vi "pick_point.vi"(4 "Modelview Matrix":sgl[][](array[numeric]), 6 "Projection Matrix":sgl[][](array[numeric]), 7 "Vertex Array":cluster{"X":sgl, "Y":sgl, "Z":sgl}[](array[cluster]), 8 "Translate By":T2, 9 "Scale By":T2, 10 "Point":cluster{"X":i32, "Y":i32}={"X"=2, "Y"=2}, 11 "ContentBounds":T1) -> (0 "Hit Any Point?":bool, 1 "Actual Ouput Coordinate":T2, 2 "Up Vect":T2, 3 "Forward Vect":T2)   [LabVIEW 2020, in "3DPC_SurfacePlot.xctl"]
uses:
  <vilib>/Native 3D Graph/xcontrol/3DPC_SurfacePlot.xctl
  <vilib>/Native 3D Graph/typedefs/vector.ctl
  <vilib>/Utility/miscctls.llb/LVBoundsTypeDef.ctl
  <vilib>/Analysis/baseanly.llb/A x Vector.vi
  <vilib>/Analysis/baseanly.llb/Real Inverse Matrix.vi
  <vilib>/Analysis/NI_AALBase.lvlib
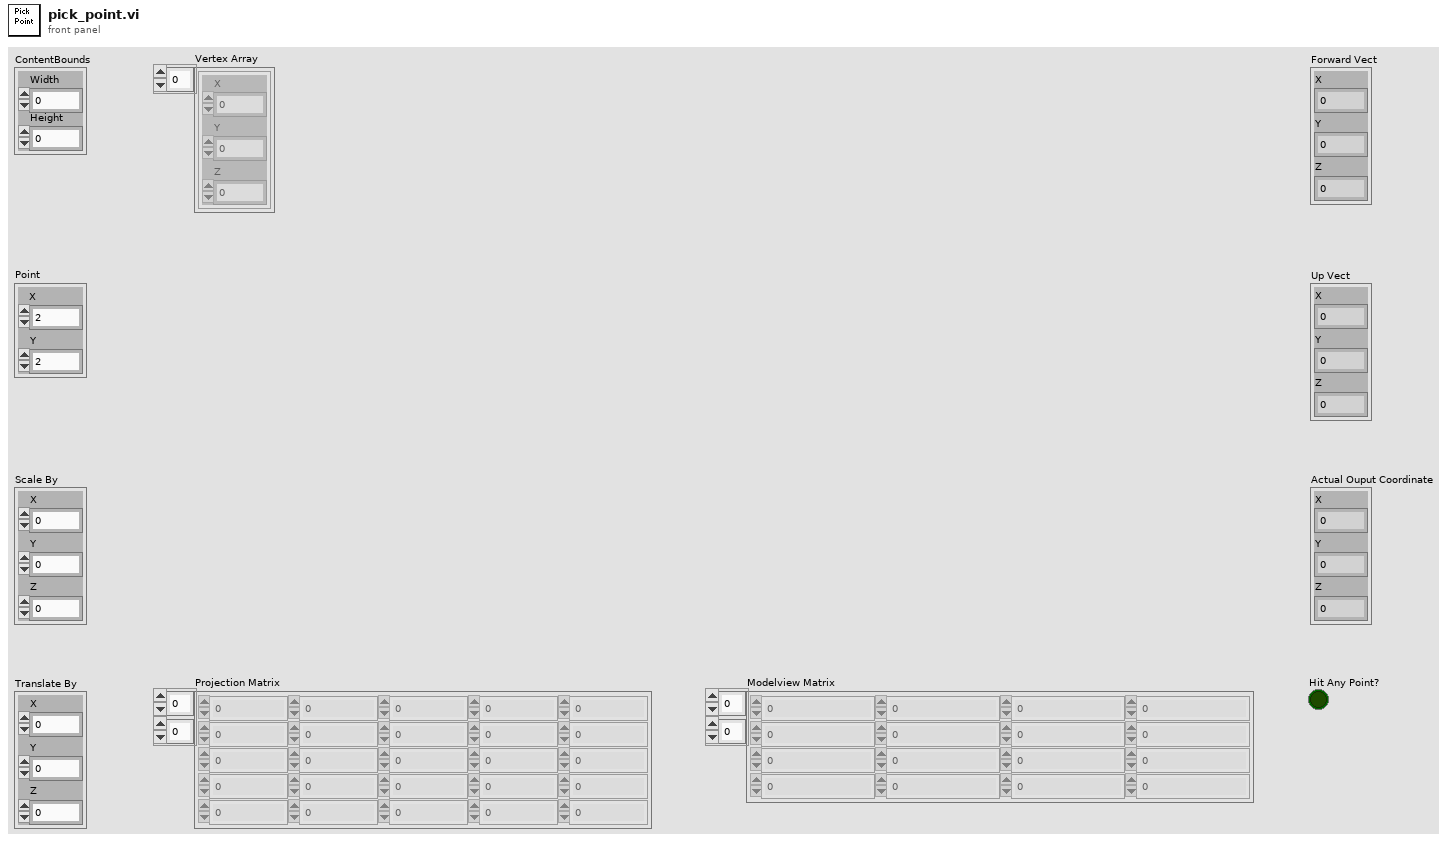
[diagram p1: front panel]
types:
  T1 = typedef "LVBoundsTypeDef.ctl" = cluster{"Width":u32, "Height":u32}
  T2 = typedef "3DPC_SurfacePlot.xctl/vector.ctl" = cluster{"X":sgl, "Y":sgl, "Z":sgl}
  T3 = cluster{"Real Matrix Element":dbl, "Real Matrix Element":dbl, "Real Matrix Element":dbl}[]
  T4 = cluster{"Real Matrix Element":i32, "Real Matrix Element":i32, "Real Matrix Element":i32}
  T5 = typedef "NI_Matrix.lvlib/RealMatrix.ctl" = dbl[][]
  T6 = cluster{"A x Vector[0]":dbl, "A x Vector[1]":dbl, "A x Vector[2]":dbl}
  T7 = cluster{cluster{"A x Vector[0]":dbl, "A x Vector[1]":dbl, "A x Vector[2]":dbl}, cluster{"A x Vector[0]":dbl, "A x Vector[1]":dbl, "A x Vector[2]":dbl}}
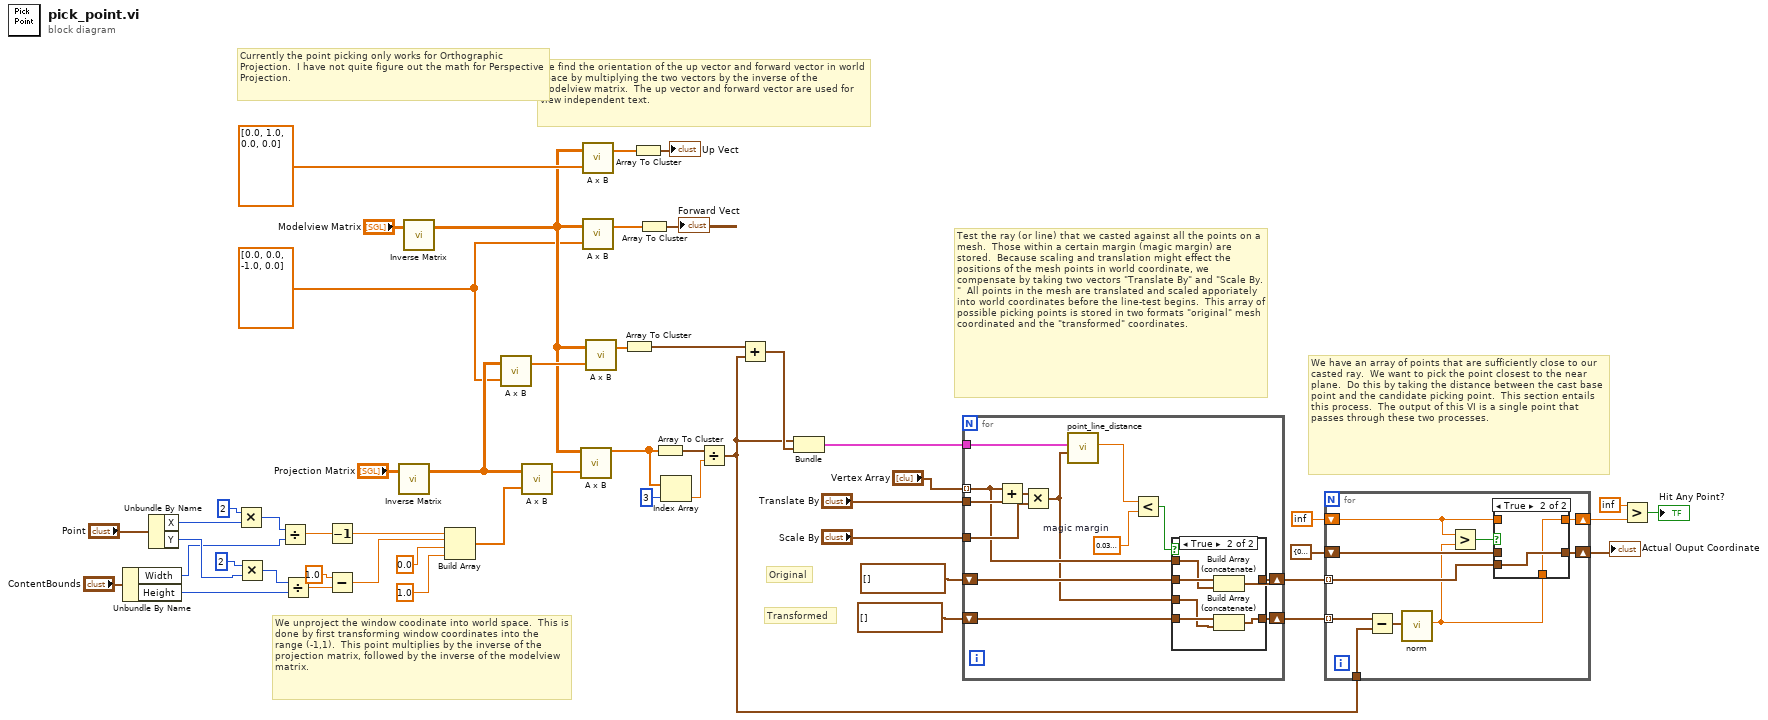
[diagram p0: block diagram]
diagram:
  w13 = dbl[] [0.0, 0.0, -1.0, 0.0]
  # "We have an array of points that are sufficiently close to our casted ray.  We want to pick the point closest to the near plane.  Do this by taking the distance between the cast base point and the candidate picking point.  This section entails this process.  The output of this VI is a single point that passes through these two processes."
  # "Test the ray (or line) that we casted against all the points on a mesh.  Those within a certain margin (magic margin) are stored.  Because scaling and translation might effect the positions of the mesh points in world coordinate, we compensate by taking two vectors \"Translate By\" and \"Scale By.\"  All points in the mesh are translated and scaled apporiately into world coordinates before the line-test begins.  This array of possible picking points is stored in two formats \"original\" mesh coordinated and the \"transformed\" coordinates."
  # "We find the orientation of the up vector and forward vector in world space by multiplying the two vectors by the inverse of the modelview matrix.  The up vector and forward vector are used for view independent text."
  # "We unproject the window coodinate into world space.  This is done by first transforming window coordinates into the range (-1,1).  This point multiplies by the inverse of the projection matrix, followed by the inverse of the modelview matrix."
  # "Currently the point picking only works for Orthographic Projection.  I have not quite figure out the math for Perspective Projection."
  # "Original"
  # "Transformed"
  n1 = Unbundle By Name("ContentBounds") -> ("Width"=w2:u32, "Height"=w1:u32)
  n2 = Unbundle By Name("Point") -> ("X"=w4:i32, "Y"=w3:i32)
  n3 = Multiply(x=2 ("y"), y=w4) -> (x*y=w51:i32)
  n4 = Multiply(x=2 ("y"), y=w3) -> (x*y=w49:i32)
  n5 = Divide(x=w51, y=w2) -> (x/y=w50:dbl)
  n6 = Divide(x=w49, y=w1) -> (x/y=w37:dbl)
  n7 = Decrement(x=w50) -> (x-1=w38:dbl)
  n8 = Subtract(x=1.0, y=w37) -> (x-y=w36:dbl)
  n9 = call-poly <vilib>:"Inverse Matrix.vi"("Input Matrix"="Projection Matrix") -> ("Inverse Matrix"=w18:T5)  [unwired: 1 in, 1 out]
  n10 = call-poly <vilib>:"Inverse Matrix.vi"("Input Matrix"="Modelview Matrix") -> ("Inverse Matrix"=w16:T5)  [unwired: 1 in, 1 out]
  n11 = Build Array(w38, w36, 0.0 ("x"), 1.0 ("element")) -> (w23:dbl[])
  n12 = call-poly <vilib>:"A x B.vi"("Vector"=w13, "A"=w18) -> ("A x Vector"=w17:dbl[])  [unwired: 1 out]
  n13 = call-poly <vilib>:"A x B.vi"("Vector"=w23, "A"=w18) -> ("A x Vector"=w46:dbl[])  [unwired: 1 out]
  n14 = call-poly <vilib>:"A x B.vi"("Vector"=w46, "A"=w16) -> ("A x Vector"=w45:dbl[])  [unwired: 1 out]
  n15 = call-poly <vilib>:"A x B.vi"("Vector"=dbl[] [0.0, 1.0, 0.0, 0.0], "A"=w16) -> ("A x Vector"=w20:dbl[])  [unwired: 1 out]
  n16 = call-poly <vilib>:"A x B.vi"("Vector"=w13, "A"=w16) -> ("A x Vector"=w34:dbl[])  [unwired: 1 out]
  n17 = call-poly <vilib>:"A x B.vi"("Vector"=w17, "A"=w16) -> ("A x Vector"=w15:dbl[])  [unwired: 1 out]
  n18 = Array To Cluster(array=w15) -> (cluster=w14:T6)
  n19 = Array To Cluster(array=w20) -> (cluster=→"Up Vect":T6)
  n20 = Array To Cluster(array=w34) -> (cluster=→"Forward Vect":T6)
  n21 = Array To Cluster(array=w45) -> (cluster=w43:T6)
  n22 = Index Array(array=w45, index=3) -> (element=w42:dbl)
  n23 = Divide(x=w43, y=w42) -> (x/y=w11:T6)
  n24 = Add(x=w14, y=w11) -> (x+y=w33:T6)
  n25 = Bundle(w11, w33) -> (w32:T7)  [unwired: 1 out]
  n26 = for {
    tunnel: "Vertex Array" -> [w58] mode=indexing
    tunnel: "Scale By" -> [w62]
    tunnel: "Translate By" -> [w63]
    tunnel: w32 -> [w60]
    shift-right: [w54] -> w29
    shift-left: T3 [] -> [w57]
    shift-right: [w53] -> w28
    shift-left: T3 [] -> [w55]
    w59 = sgl 0.04  # magic margin
    n27 = Add(x=w58, y=w63) -> (x+y=w64:T2)
    n28 = Multiply(x=w64, y=w62) -> (x*y=w56:T2)
    n29 = call <vilib>:"point_line_distance.vi"("Point"=w56, "Line"=w60) -> ("Distance"=w61:sgl)  [unwired: 9 out]
    n30 = Less?(x=w61, y=w59) -> (x < y?=w65:bool)
    n31 = case shown="True" w65 {
      tunnel: w58 -> [_ w72]
      tunnel: w57 -> [w67 w73]
      tunnel: w56 -> [_ w69]
      tunnel: w55 -> [w66 w70]
      tunnel: [w67 w71] -> w54
      tunnel: [w66 w68] -> w53
      frame False {
      }
      frame True {
        n32 = Build Array (concatenate)(w73, w72) -> (w71:T3)
        n33 = Build Array (concatenate)(w70, w69) -> (w68:T3)
      }
    }
  }
  n34 = for {
    tunnel: w29 -> [w75] mode=indexing
    tunnel: w28 -> [w83] mode=indexing
    shift-right: [w78] -> w9
    shift-left: T4 {"Real Matrix Element"=0, "Real Matrix Element"=0, "Real Matrix Element"=0} -> [w79]
    shift-right: [w76] -> w25
    shift-left: inf -> [w77]
    tunnel: w11 -> [w82]
    n35 = Subtract(x=w83, y=w82) -> (x-y=w81:cluster{dbl, dbl, dbl})
    n36 = call <vilib>:"norm.vi"("Vector"=w81) -> ("Norm"=w74:sgl)  [unwired: 10 out]
    n37 = Greater?(x=w77, y=w74) -> (0:w80:bool)
    n38 = case shown="True" w80 {
      tunnel: w79 -> [w85 _]
      tunnel: [w85 w87] -> w78
      tunnel: w77 -> [w84 _]
      tunnel: [w84 w86] -> w76
      tunnel: w75 -> [_ w87]
      tunnel: w74 -> [_ w86]
      frame False {
      }
      frame True {
      }
    }
  }
  "Actual Ouput Coordinate" <- w9
  n39 = Greater?(x=inf, y=w25) -> (0:→"Hit Any Point?":bool)
